vi "TEST - Array Dim(s) from TD.vi"(8 "error in (no error)":errorcluster) -> (0 "error out":errorcluster, 2 "pass":bool)   [LabVIEW 2020, in "test_openg_array.lvlib"]
uses:
  source/library/Type Descriptor.ctl
  source/library/Type Descriptor Enumeration.ctl
  test_openg_array.lvlib
  <userlib>/_OpenG.lib/error/error.llb/openg_error.lvlib
  source/library/openg_variant.lvlib
panel:
  out "Failures":T3(array[cluster]) {"type" format="%.0x"}
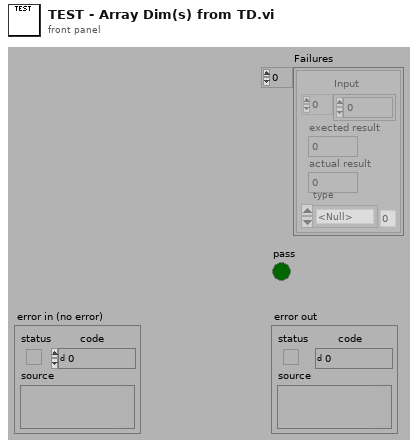
[diagram p1: front panel]
types:
  T1 = typedef "openg_variant.lvlib/Type Descriptor.ctl" = i16[]
  T2 = typedef "openg_variant.lvlib/Type Descriptor Enumeration.ctl" = enum8{"<Null>", "I8", "I16", "I32", "I64", "U8", "U16", "U32", "U64", "SGL", "DBL", "EXT", "CSG", "CDB", "CXT", "0x0F", "0x10", "0x11", "0x12", "0x13", "0x14", "Enum U8", "Enum U16", "Enum U32", "Enum U64", "SGL PQ", "DBL PQ", "EXT PQ", "CSG PQ", "CDB PQ", "CXT PQ", "0x1F", "0x20", "Boolean", "0x22", "0x23", "0x24", "0x25", "0x26", "0x27", "0x28", "0x29", "0x2A", "0x2B", "0x2C", "0x2D", "0x2E", "0x2F", "String", "0x31", "Path", "Pict", "0x34", "0x35", "0x36", "DAQ", "0x38", "0x39", "0x3A", "0x3B", "0x3C", "0x3D", "0x3E", "0x3F", "Array", "0x41", "0x42", "0x43", "0x44", "0x45", "0x46", "0x47", "0x48", "0x49", "0x4A", "0x4B", "0x4C", "0x4D", "0x4E", "0x4F", "Cluster", "0x51", "0x52", "Variant", "Waveform", "0x55", "0x56", "0x57", "0x58", "0x59", "0x5A", "0x5B", "0x5C", "0x5D", "0x5E", "Fixed Point", "0x60", "0x61", "0x62", "0x63", "0x64", "0x65", "0x66", "0x67", "0x68", "0x69", "0x6A", "0x6B", "0x6C", "0x6D", "0x6E", "0x6F", "Refnum", "0x71", "0x72", "Set Collection", "Map Collection"}
  T3 = cluster{"Input":T1, "exected result":i32, "actual result":i32, "type":T2}[]
  T4 = typedef "openg_variant.lvlib/Type Descriptor Header.ctl" = cluster{"length":u16, "private":u8, "type":T2, "# elements":u16}
  T5 = cluster{"Input":T1, "exected result":i32, "actual result":i32, "type":T2}
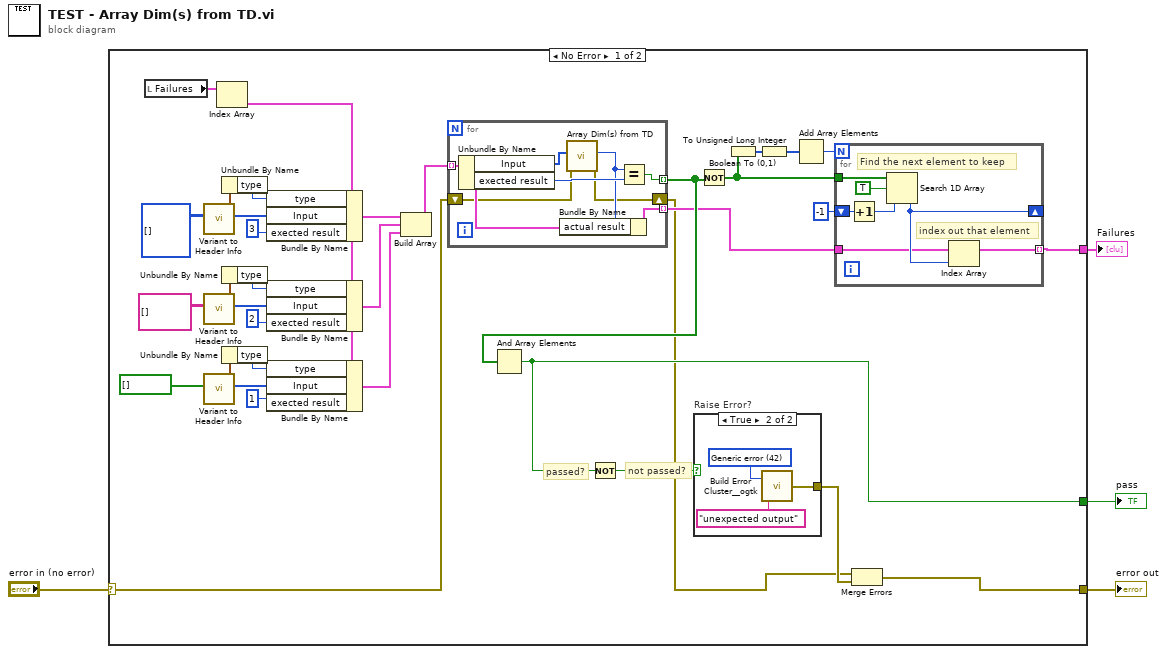
[diagram p0: block diagram]
diagram:
  n1 = case shown="No Error" "error in (no error)" {
    selector: "error in (no error)" -> [w8 w58]
    tunnel: [w36 _] -> w4
    tunnel: [w39 w58] -> w2
    tunnel: [w28 _] -> w1
    frame No Error {
      # "not passed?"
      # "passed?"
      n2 = local read "Failures"() -> (w6:T3)
      n3 = call "Variant to Header Info.vi"("Variant"=i32[][][] []) -> ("Type Descriptor Header"=w22:T4, "Type Descriptor"=w26:T1)  [unwired: 3 in, 1 out]
      n4 = call "Variant to Header Info.vi"("Variant"=string[][] []) -> ("Type Descriptor Header"=w19:T4, "Type Descriptor"=w17:T1)  [unwired: 3 in, 1 out]
      n5 = call "Variant to Header Info.vi"("Variant"=bool[] []) -> ("Type Descriptor Header"=w15:T4, "Type Descriptor"=w11:T1)  [unwired: 3 in, 1 out]
      n6 = Index Array(array=w6) -> (element=w5:T5)  [unwired: 1 in]
      n7 = Unbundle By Name(w22) -> ("type"=w21:T2)
      n8 = Unbundle By Name(w19) -> ("type"=w20:T2)
      n9 = Unbundle By Name(w15) -> ("type"=w12:T2)
      n10 = Bundle By Name(cluster=w5, "type"=w21, "Input"=w26, "exected result"=3) -> (w24:T5)
      n11 = Bundle By Name(cluster=w5, "type"=w20, "Input"=w17, "exected result"=2) -> (w14:T5)
      n12 = Bundle By Name(cluster=w5, "type"=w12, "Input"=w11, "exected result"=1) -> (w13:T5)
      n13 = Build Array(w24, w14, w13) -> (w23:T3)
      n14 = for {
        tunnel: w23 -> [w51] mode=indexing
        tunnel: [w54] -> w30 mode=indexing
        tunnel: [w52] -> w29 mode=indexing
        shift-right: [w47] -> w7
        shift-left: w8 -> [w48]
        n15 = Unbundle By Name(w51) -> ("Input"=w50:T1, "exected result"=w53:i32)
        n16 = call "Array Dim(s) from TD.vi"("error in (no error)"=w48, "Array Type Descriptor"=w50) -> ("error out"=w47:errorcluster, "N dims"=w49:u32)  [unwired: 8 in]
        n17 = Bundle By Name(cluster=w51, "actual result"=w49) -> (w52:T5)
        n18 = Equal?(x=w49, y=w53) -> (x = y?=w54:bool)
      }
      n19 = And Array Elements(Boolean array=w30) -> (logical AND=w36:bool)
      n20 = Not(x=w36) -> (.not. x?=w37:bool)
      n21 = case "Raise Error?" shown="True" w37 {
        tunnel: [_ w55] -> w38
        frame False {
        }
        frame True {
          w56 = 42 items=["No error", "Argument error", "Memory is full", "Out of zone", "End of file", "File already open", "Generic file I/O error", "File not found", "File permission error", "Disk is full", "Duplicate path", "Too many files open", "System feature not enabled", "Resource file not found", "Cannot add resource", "Resource not found", "Image not found", "Image memory error", "Pen does not exist", "Config type invalid", "Config token not found", "Config parse error", "Config memory error", "Bad external code format", "Bad external code offset", "External code not present", "Null window", "Destroy window error", "Null menu", "Print aborted", "Bad print record", "Print driver error", "Windows error during printing", "Memory error during printing", "Print dialog error", "Generic print error", "Invalid device refnum", "Device not found", "Device parameter error", "Device unit error", "Cannot open device", "Device call aborted", "Generic error", "Cancelled by user", "Object ID too low", "Object ID too high", "Object not in heap", "Unknown heap", "Unknown object (invalid DefProc)", "Unknown object (DefProc not in table)", "Message out of range", "Invalid (null) method", "Unknown message", "Manager call not supported", "Bad address", "Network operation in progress", "Network operation timed out", "Connection is busy", "Network attribute not supported", "Network error", "Address in use", "System out of memory", "Connection aborted", "Connection refused", "Not connected", "Already connected", "Connection closed", "Initialization error (interapplication manager)", "Bad occurrence", "Wait on unbound occurrence handler", "Occurrence queue overflow", "Datalog type conflict", "Unused", "Unrecognized type (interapplication manager)", "Memory corrupt", "Failed to make temporary DLL", "Old CIN version", "Drag socket not found", "Failed to load drop-object", "Failed to register OLE object", "Failed to release OLE object", "Format specifier type mismatch", "Unknown format specifier", "Too few format specifiers", "Too many format specifiers", "Scan failed", "Newer CIN version", "Error converting to variant", "Runtime menu error", "Password tampered", "Variant attribute not found", "Incompatible variant data type", "Event data is not available", "Event Store is not present", "Occurrence is not found", "Event Queue is not created", "Event info is not available", "Refnum passed is NULL", "Error retrieving Class GUID", "Error retrieving CoClass GUID", "Error retrieving TypeLib GUID.", "Bad built application magic bytes.", "Specific driver is different from the specific driver associated with the Logical Name.", "There is no session opened to the class driver.", "Max Error", "MAX - Error with config objects", "MAX - Error loading configuration", "MAX - Group not supported"]
          n22 = call <userlib>:"Build Error Cluster__ogtk.vi"("String to Prepend to source (\"\")"="unexpected output" ("String to Prepend to source (\"\")"), "code"=w56) -> ("error out"=w55:errorcluster)
        }
      }
      n23 = Not(x=w30) -> (.not. x?=w32:bool[])
      n24 = Boolean To (0,1)(Boolean=w32) -> (0, 1=w33:i16[])
      n25 = To Unsigned Long Integer(number=w33) -> (unsigned 32bit integer=w31:u32[])
      n26 = Add Array Elements(numeric array=w31) -> (sum=w34:u32)
      n27 = for {
        N: w34 -> [_]
        tunnel: w29 -> [w42]
        tunnel: w32 -> [w46]
        shift-right: [w43] -> _
        shift-left: -1 ("start index (0)") -> [w44]
        tunnel: [w41] -> w28 mode=indexing
        # "index out that element"
        # "Find the next element to keep"
        n28 = Increment(x=w44) -> (x+1=w40:i32)
        n29 = Search 1D Array(1D array=w46, element=TRUE, start index (0)=w40) -> (index of element=w43:i32)
        n30 = Index Array(array=w42, index=w43) -> (element=w41:T5)
      }
      n31 = Merge Errors(w7, w38) -> (w39:errorcluster)
    }
    frame Error {
    }
  }
  "pass" <- w4
  "error out" <- w2
  "Failures" <- w1
